vi "Main.vi"() -> ()   [LabVIEW 2020, in "DAQ AO SFP.lvlib"]
uses:
  DAQ AO SFP.lvlib
  WaveGen/Shape.ctl
  UI Refs.ctl
  <extravilib>/ChannelInstances/Flex-t'DAQmx AO.lvlib-Status.ctl'/Instantiate.vi
  <extravilib>/ChannelInstances/Flex-t'DAQmx AO.lvlib-Action.ctl'/Instantiate.vi
  <extravilib>/ChannelInstances/Flex-t'DAQmx AO.lvlib-Params.ctl'/Instantiate.vi
  <extravilib>/ChannelInstances/Flex-t'WaveGen.lvlib-Gen Action.ctl'/Instantiate.vi
  <extravilib>/ChannelInstances/Flex-t'WaveGen.lvlib-Gen Params.ctl'/Instantiate.vi
  <extravilib>/ChannelInstances/Flex-a[.](wfm(dbl))/Instantiate.vi
  WaveGen/WaveGen.lvlib
  DAQmx AO/DAQmx AO.lvlib
  <extravilib>/ChannelInstances/Flex-a[.](wfm(dbl)).lvlib
panel:
  out "Period":dbl=1.4048832999978913 format="%#_6f"
  out "Active":bool
  out "Valid":bool=TRUE
  in  "Channels":tag="SimAO/ao0:1"
  out "Graph":waveform(dbl)[](graph)
  in  "Offset 2":dbl(slide) scale=-2.5..2.5
  in  "Amplitude 2":dbl(slide)=5.0 scale=0.0..5.0
  in  "Frequency 2":dbl(slide)=35.05 scale=0.1..1000.0
  in  "Shape 2":T1
  in  "Count":dbl=10000.0 format="%#_3p"
  in  "Rate":dbl=100000.0 format="%_3p"
  in  "Start":bool
  in  "Offset":dbl(slide)=0.05 scale=-2.5..2.5
  in  "Amplitude":dbl(slide)=5.0 scale=0.0..5.0
  in  "Frequency":dbl(slide)=34.95 scale=0.1..1000.0
  in  "Shape":T1
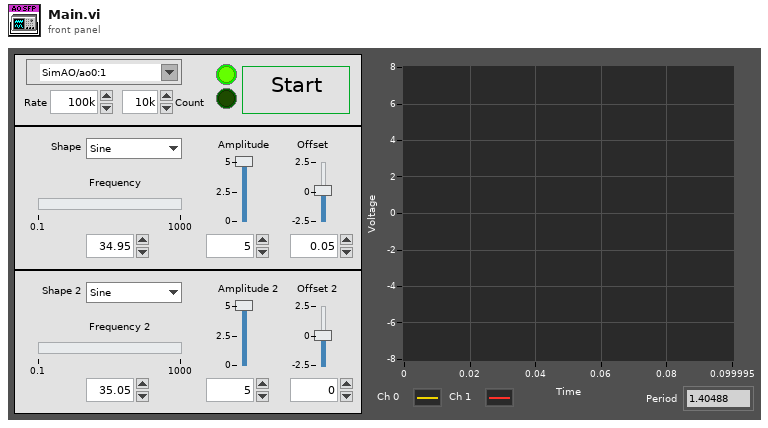
[diagram p1: front panel]
types:
  T1 = typedef "WaveGen.lvlib/Shape.ctl" = enum16{"Sine", "Square", "Triangle", "Saw"}
  T2 = typedef "DAQ AO SFP.lvlib/UI Refs.ctl" = cluster{"VI":refnum<vi>, "Rate":refnum<vi>, "Count":refnum<vi>, "Start":refnum<vi>, "Shape":refnum<vi>, "Frequency":refnum<vi>, "Amplitude":refnum<vi>, "Offset":refnum<vi>, "Shape 2":refnum<vi>, "Frequency 2":refnum<vi>, "Amplitude 2":refnum<vi>, "Offset 2":refnum<vi>, "Channels":refnum<vi>, "Valid":refnum<vi>, "Active":refnum<vi>}
  T3 = typedef "Flex-t'WaveGen.lvlib-Gen Action.ctl'.lvlib/))Channel.ctl" = refnum<queue>
  T4 = typedef "Flex-t'WaveGen.lvlib-Gen Params.ctl'.lvlib/))Channel.ctl" = refnum<queue>
  T5 = typedef "Flex-t'DAQmx AO.lvlib-Params.ctl'.lvlib/))Channel.ctl" = refnum<queue>
  T6 = typedef "Flex-t'DAQmx AO.lvlib-Action.ctl'.lvlib/))Channel.ctl" = refnum<queue>
  T7 = typedef "Flex-a[.](wfm(dbl)).lvlib/))Channel.ctl" = refnum<queue>
  T8 = typedef "Flex-t'DAQmx AO.lvlib-Status.ctl'.lvlib/))Channel.ctl" = refnum<queue>
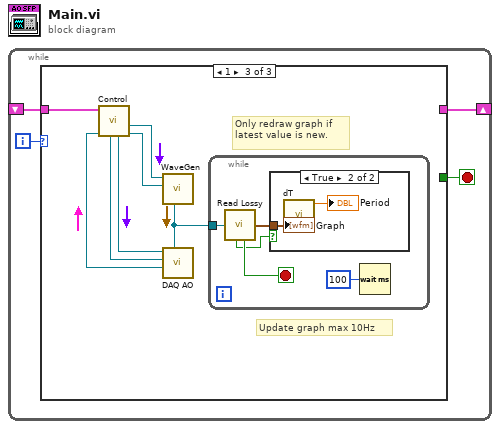
[diagram p0: block diagram]
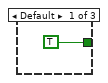
[diagram p2: hidden frame]
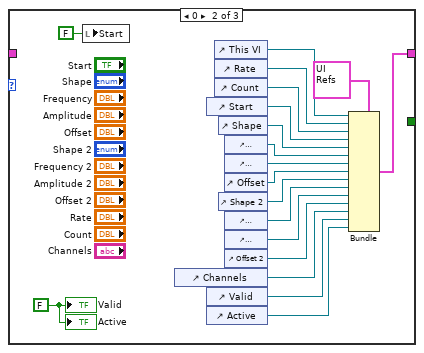
[diagram p3: hidden frame]
diagram:
  n1 = while {
    shift-right: [w2] -> _
    shift-left: _ -> [w4]
    i -> [w3]
    stop <- w1 stop-if-true
    n2 = case shown="1" w3 {
      tunnel: w4 -> [_ _ w30]
      tunnel: [_ w11 _] -> w2
      tunnel: [TRUE _ _] -> w1
      frame Default {
      }
      frame 0 {
        w6 = FALSE ("Valid")
        n3 = local write "Start"(FALSE ("Start")) -> ()
        n4 = control-ref of="Channels"() -> (w24:refnum<vi>)
        n5 = control-ref of="Start"() -> (w16:refnum<vi>)
        n6 = control-ref of="Valid"() -> (w9:refnum<vi>)
        n7 = control-ref of="Active"() -> (w8:refnum<vi>)
        n8 = control-ref of="This VI"() -> (w10:refnum<vi>)
        n9 = control-ref of="Rate"() -> (w18:refnum<vi>)
        n10 = control-ref of="Count"() -> (w17:refnum<vi>)
        n11 = control-ref of="Shape"() -> (w15:refnum<vi>)
        n12 = control-ref of="Shape 2"() -> (w20:refnum<vi>)
        n13 = control-ref of="Frequency"() -> (w14:refnum<vi>)
        n14 = control-ref of="Amplitude"() -> (w13:refnum<vi>)
        n15 = control-ref of="Offset"() -> (w19:refnum<vi>)
        n16 = control-ref of="Frequency 2"() -> (w21:refnum<vi>)
        n17 = control-ref of="Amplitude 2"() -> (w22:refnum<vi>)
        n18 = control-ref of="Offset 2"() -> (w23:refnum<vi>)
        n19 = Bundle(cluster=T2 {"VI"=refnum, "Rate"=refnum, "Count"=refnum, "Start"=refnum, "Shape"=refnum, "Frequency"=refnum, "Amplitude"=refnum, "Offset"=refnum, "Shape 2"=refnum, "Frequency 2"=refnum, "Amplitude 2"=refnum, "Offset 2"=refnum, "Channels"=refnum, "Valid"=refnum, "Active"=refnum}, "VI"=w10, "Rate"=w18, "Count"=w17, "Start"=w16, "Shape"=w15, "Frequency"=w14, "Amplitude"=w13, "Offset"=w19, "Shape 2"=w20, "Frequency 2"=w21, "Amplitude 2"=w22, "Offset 2"=w23, "Channels"=w24, "Valid"=w9, "Active"=w8) -> (w11:T2)
        "Valid" <- w6
        "Active" <- w6
      }
      frame 1 {
        # "Only redraw graph if latest value is new."
        # "Update graph max 10Hz"
        n20 = call "Control.vi"("DAQ Status"=w25, "UI Refs"=w30) -> ("WaveGen Action"=w28:T3, "WaveGen Params"=w29:T4, "DAQ Params"=w27:T5, "DAQ Action"=w26:T6)  [unwired: 6 in]
        n21 = call "WaveGen.vi"("Action"=w28, "Params"=w29) -> ("Signals"=w31:T7)  [unwired: 9 in]
        n22 = call "DAQ AO.vi"("Signals"=w31, "Action"=w26, "Params"=w27) -> ("Status"=w25:T8)  [unwired: 8 in]
        n23 = while {
          tunnel: w31 -> [w36]
          stop <- w35 stop-if-true
          n24 = call <extravilib>:"Read Lossy.vi"("FlexChannel"=w36) -> ("New Value?"=w32:bool, "Value"=w34:waveform(dbl)[], "Closed?"=w35:bool)  [unwired: 4 in, 2 out]
          n25 = case shown="True" w32 {
            tunnel: w34 -> [_ w38]
            frame False {
            }
            frame True {
              n26 = call "dT.vi"() -> ("Period"=→"Period":dbl)  [unwired: 11 in]
              "Graph" <- w38
            }
          }
          n27 = Wait (ms)(milliseconds to wait=u32 100) -> ()  [unwired: 1 out]
        }
      }
    }
  }
